vi "_HC_PM_and_temp.vi"(9 "PMavg":dbl=10.0, 10 "Bias_LO_equip":T1={"Node address"=19, "CAN Interface"="CAN1", "Cartridge band"=10, "Slave Node in"={"Address"=19, "Serial Number"=[16, 71, 55, 76, 1, 8, 0, -15]}, "ObjHandle out"=176554048, "POL"=1, "sb"=1, "GPIB_SM (SIS S,V)"="24", "GPIB_DMM (SIS I)"="22", "GPIB_SM (MAG I) "="25", "GPIB_SG(LO)"="19", "GPIB_PW (PAMP) "="6", "GPIB_TMP1(8ch)"="12", "GPIB_TMP2(2ch)  "="13", "WCA_avg"=10, "Rsen"=10.0, "BiasModule"=1, "LOModule "=5, "WCA_LO_FREQ_SET"={"YTO Low freq. [GHz]"=14.42, "YTO High freq. [GHz]"=17.7, "Kvco"=1, "Lock Pol."=0, "SET LO FREQ"=96.22222, "Multiplier"=6.0, "YTO (HEX)"=2014, "YTO ( FREQ)"=16.033167, "NULL PLL INTEGRATOR"=FALSE}, "Res for"=0} {"Res for" items=["none", "series res", "parallel res"]; "WCA_LO_FREQ_SET"."YTO ( FREQ)" min=25 max=150 step=0.0001 format="%.3f"; "WCA_LO_FREQ_SET"."Multiplier" min=3 max=6 step=3; "WCA_LO_FREQ_SET"."SET LO FREQ" min=25 max=150 step=0.0001 format="%.3f"; "WCA_LO_FREQ_SET"."Lock Pol." items=["Lower", "Upper"]; "WCA_LO_FREQ_SET"."Kvco" items=["7.5MHz/V", "15MHz/V"]; "WCA_LO_FREQ_SET"."YTO High freq. [GHz]" format="%.3f"; "WCA_LO_FREQ_SET"."YTO Low freq. [GHz]" format="%.3f"; "LOModule" items=["Manual Gunn+PAMP"=0, "PLL GUNN+PAMP"=5, "B10Lab LO"=1, "WCA LO"=2, ""=3, "YIG発信器"=4, "none"=99]; "BiasModule" items=["B10Lab Bias"=0, "WCA BiasModule"=1, "none"=99]; "Slave Node in"."Serial Number" format="%.0x"; "Slave Node in"."Address" format="%.0x"; "Cartridge band" max=10 step=1; "Node address" format="%.0x"}, 11 "Control":T2={"GPIB_ATT"="28", "6501Dev#"=1, "GPIB_SP"="18", "GPIB_PM"="13", "GPIB_DSA"="11", "GPIB_DMM (TPD)"="23", "GPIB_MPI"="2", "mortor設定"=[{"Axis"=0, "ID"=0, "HIspeed"=200.0, "LOspeed"=100.0, "ACCEL(ms)"=100.0, "Sratio"=50.0, "フリーラン\n"=FALSE, "文字列"="DSB HOT/COLD"}, {"Axis"=1, "ID"=0, "HIspeed"=4.0, "LOspeed"=4.0, "ACCEL(ms)"=100.0, "Sratio"=50.0, "フリーラン\n"=TRUE, "文字列"="SubMM Att"}, {"Axis"=0, "ID"=0, "HIspeed"=200.0, "LOspeed"=100.0, "ACCEL(ms)"=100.0, "Sratio"=50.0, "フリーラン\n"=TRUE, "文字列"="MPI Port1"}, {"Axis"=1, "ID"=0, "HIspeed"=200.0, "LOspeed"=100.0, "ACCEL(ms)"=100.0, "Sratio"=50.0, "フリーラン\n"=TRUE, "文字列"="MPI Port2"}], "DATAパス"=path "C:/Documents and Settings/?澤佳?/デスクトップ/data/プロトカ?トリッジ/100811_protC4-5/100904_P1_WCA_YIG", "DBパス "=path "Z:/band10/Labview_ALMA/MIX95/test", "comment"="100904_P1", "ColdCarts"="003601", "Th"=295.0, "Tc"=77.0, "Set_SIS_volt"=2.056451612903226, "Offset"=0.0, "control"=0, "FreqLO"=866.0, "Set_Mag_Cur"=800.0, "MPI offset(mm)"=22.986, "HOT/COLD"=0} {"HOT/COLD" items=["DSB", "SBR (Cart.)", "GainComp", "SBR (MIX)"]; "control" items=["CLOSE LOOP", "OPEN LOOP", "Not Control"]}) -> (3 "文字列":string="298.140000,297.760000,298.730000,304.990000,4.072000,4.151000,15.042000,80.446000,-19.064756,-17.597972,-30.625485,")   [LabVIEW 2017]
panel:
  # "LO freq. [GHz]"
  # "YTO LOW\n/High Freq."
  # "ZERO Intgrtr"
  # "Node Address"
  # "Serial Number"
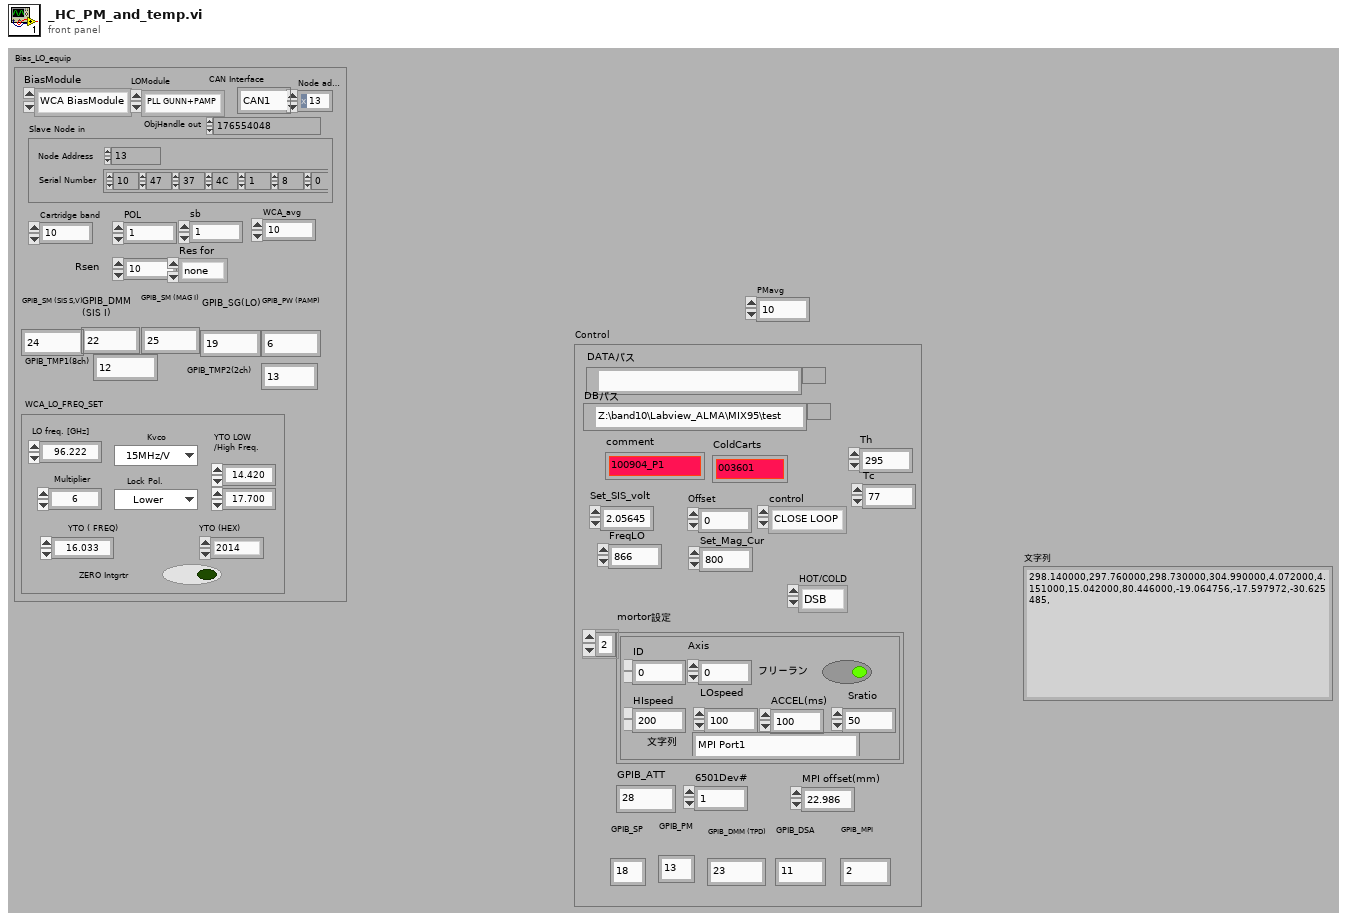
[diagram p1: front panel]
types:
  T1 = cluster{"Node address":u16, "CAN Interface":string, "Cartridge band":u32, "Slave Node in":cluster{"Address":i16, "Serial Number":i8[]}, "ObjHandle out":u32, "POL":u32, "sb":u32, "GPIB_SM (SIS S,V)":string, "GPIB_DMM (SIS I)":string, "GPIB_SM (MAG I) ":string, "GPIB_SG(LO)":string, "GPIB_PW (PAMP) ":string, "GPIB_TMP1(8ch)":string, "GPIB_TMP2(2ch)  ":string, "WCA_avg":i32, "Rsen":dbl, "BiasModule":u16, "LOModule ":u16, "WCA_LO_FREQ_SET":cluster{"YTO Low freq. [GHz]":sgl, "YTO High freq. [GHz]":sgl, "Kvco":u16, "Lock Pol.":u16, "SET LO FREQ":sgl, "Multiplier":sgl, "YTO (HEX)":u16, "YTO ( FREQ)":sgl, "NULL PLL INTEGRATOR":bool}, "Res for":u16}
  T2 = cluster{"GPIB_ATT":string, "6501Dev#":i16, "GPIB_SP":string, "GPIB_PM":string, "GPIB_DSA":string, "GPIB_DMM (TPD)":string, "GPIB_MPI":string, "mortor設定":cluster{"Axis":i16, "ID":i16, "HIspeed":dbl, "LOspeed":dbl, "ACCEL(ms)":dbl, "Sratio":dbl, "フリーラン\n":bool, "文字列":string}[], "DATAパス":path, "DBパス ":path, "comment":string, "ColdCarts":string, "Th":dbl, "Tc":dbl, "Set_SIS_volt":dbl, "Offset":dbl, "control":u16, "FreqLO":dbl, "Set_Mag_Cur":dbl, "MPI offset(mm)":dbl, "HOT/COLD":u16}
  T3 = cluster{"Axis":i16, "ID":i16, "HIspeed":dbl, "LOspeed":dbl, "ACCEL(ms)":dbl, "Sratio":dbl, "フリーラン\n":bool, "文字列":string}[]
  T4 = cluster{"Axis":i16, "ID":i16, "HIspeed":dbl, "LOspeed":dbl, "ACCEL(ms)":dbl, "Sratio":dbl, "フリーラン\n":bool, "文字列":string}
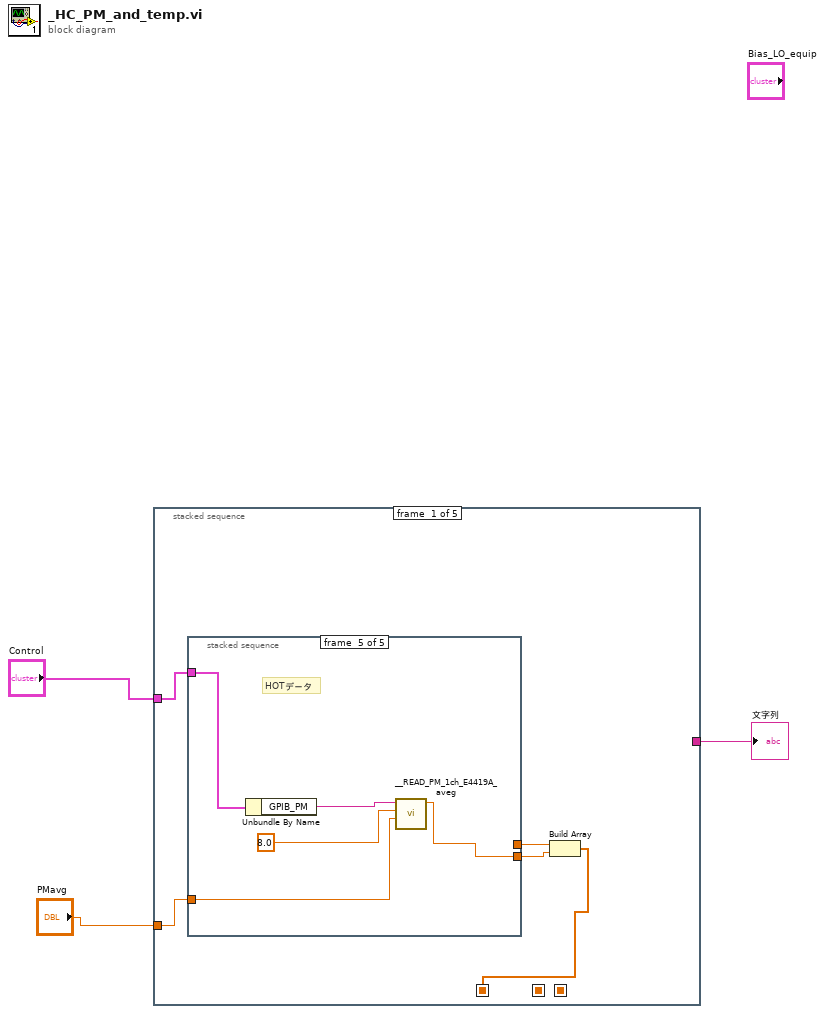
[diagram p0: block diagram]
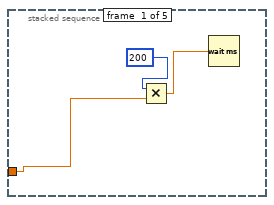
[diagram p2: hidden frame]
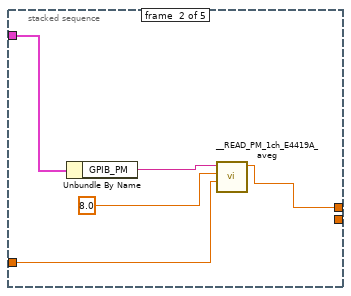
[diagram p3: hidden frame]
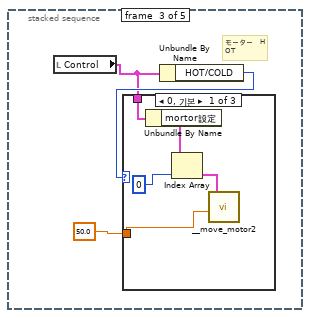
[diagram p4: hidden frame]
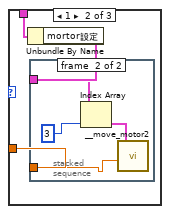
[diagram p5: hidden frame]
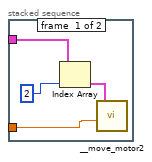
[diagram p6: hidden frame]
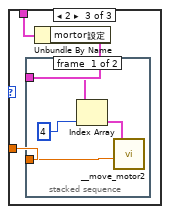
[diagram p7: hidden frame]
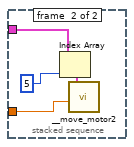
[diagram p8: hidden frame]
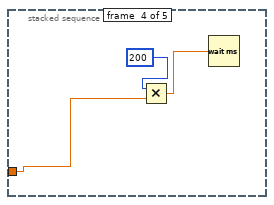
[diagram p9: hidden frame]
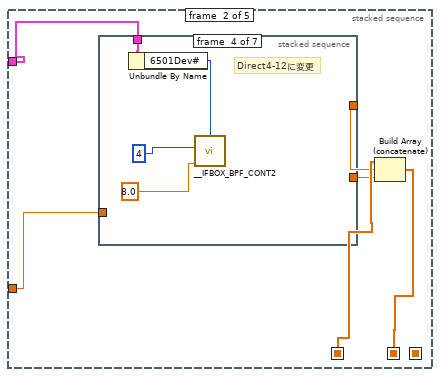
[diagram p10: hidden frame]
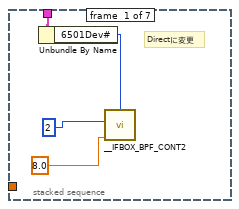
[diagram p11: hidden frame]
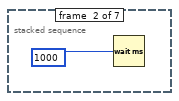
[diagram p12: hidden frame]
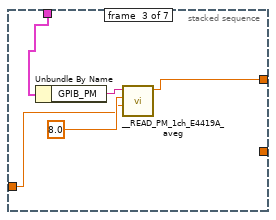
[diagram p13: hidden frame]
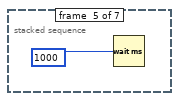
[diagram p14: hidden frame]
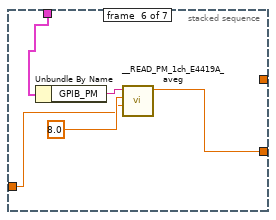
[diagram p15: hidden frame]
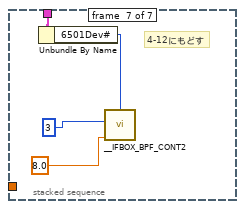
[diagram p16: hidden frame]
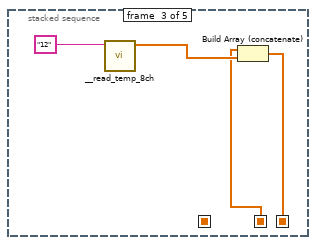
[diagram p17: hidden frame]
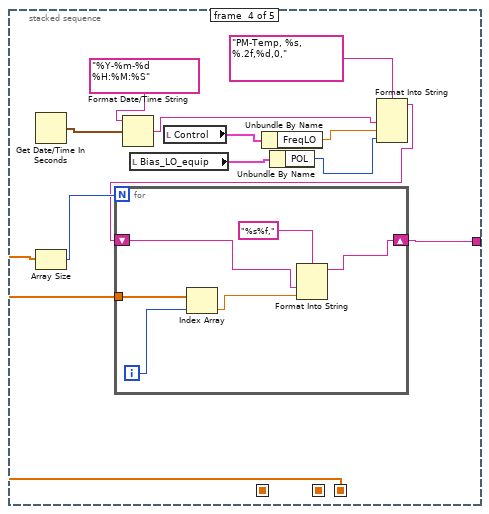
[diagram p18: hidden frame]
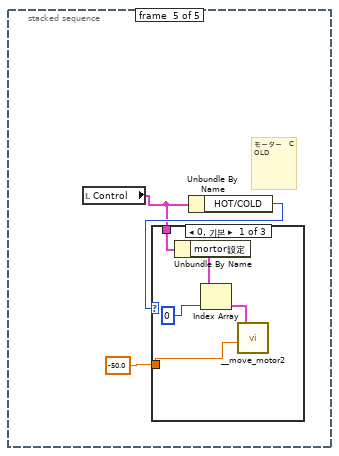
[diagram p19: hidden frame]
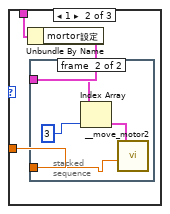
[diagram p20: hidden frame]
diagram:
  n1 = stacked-sequence {
    seq-local: [w4 _ _ _ _] -> [_ w57 _ _ _]
    seq-local: [_ w58 _ _ _] -> [_ _ w85 _ _]
    seq-local: [_ _ w86 _ _] -> [_ _ _ w89 _]
    tunnel: "Control" -> [w8 w60 _ _ _]
    tunnel: "PMavg" -> [w7 w59 _ _ _]
    tunnel: [_ _ _ w99 _] -> w1
    frame #0 {
      n2 = stacked-sequence {
        tunnel: w8 -> [_ w15 _ _ w53]
        tunnel: w7 -> [w9 w13 _ w47 w51]
        tunnel: [_ w12 _ _ _] -> w6
        tunnel: [_ _ _ _ w50] -> w5
        frame #0 {
          n3 = Multiply(x=200, y=w9) -> (x*y=w11:dbl)
          n4 = Wait (ms)(milliseconds to wait=w11) -> ()  [unwired: 1 out]
        }
        frame #1 {
          n5 = Unbundle By Name(w15) -> ("GPIB_PM"=w16:string)
          n6 = call "__READ_PM_1ch_E4419A_aveg.VI"("aveg"=w13, "frq(GHz)"=8.0, "GPIB"=w16) -> ("chA"=w12:dbl)  [unwired: 4 in]
        }
        frame #2 {
          # "モーター　HOT"
          n7 = local read "Control"() -> (w17:T2)
          n8 = Unbundle By Name(w17) -> ("HOT/COLD"=w18:u16)
          n9 = case shown="0, 기본" w18 {
            tunnel: w17 -> [w23 w27 w38]
            tunnel: 50.0 -> [w20 w25 w36]
            frame 0, Default {
              n10 = Unbundle By Name(w23) -> ("mortor設定"=w22:T3)
              n11 = Index Array(array=w22, index=0) -> (element=w21:T4)
              n12 = call "__move_motor2.vi"("Moving distance"=w20, "motor setup"=w21) -> ()  [unwired: 2 in, 2 out]
            }
            frame 1 {
              n13 = Unbundle By Name(w27) -> ("mortor設定"=w26:T3)
              n14 = stacked-sequence {
                tunnel: w26 -> [w30 w34]
                tunnel: w25 -> [w28 w32]
                frame #0 {
                  n15 = Index Array(array=w30, index=2) -> (element=w29:T4)
                  n16 = call "__move_motor2.vi"("Moving distance"=w28, "motor setup"=w29) -> ()  [unwired: 2 in, 2 out]
                }
                frame #1 {
                  n17 = Index Array(array=w34, index=3) -> (element=w33:T4)
                  n18 = call "__move_motor2.vi"("Moving distance"=w32, "motor setup"=w33) -> ()  [unwired: 2 in, 2 out]
                }
              }
            }
            frame 2 {
              n19 = Unbundle By Name(w38) -> ("mortor設定"=w37:T3)
              n20 = stacked-sequence {
                tunnel: w37 -> [w41 w45]
                tunnel: w36 -> [w39 w43]
                frame #0 {
                  n21 = Index Array(array=w41, index=4) -> (element=w40:T4)
                  n22 = call "__move_motor2.vi"("Moving distance"=w39, "motor setup"=w40) -> ()  [unwired: 2 in, 2 out]
                }
                frame #1 {
                  n23 = Index Array(array=w45, index=5) -> (element=w44:T4)
                  n24 = call "__move_motor2.vi"("Moving distance"=w43, "motor setup"=w44) -> ()  [unwired: 2 in, 2 out]
                }
              }
            }
          }
        }
        frame #3 {
          n25 = Multiply(x=200, y=w47) -> (x*y=w49:dbl)
          n26 = Wait (ms)(milliseconds to wait=w49) -> ()  [unwired: 1 out]
        }
        frame #4 {
          # "HOTデータ"
          n27 = Unbundle By Name(w53) -> ("GPIB_PM"=w54:string)
          n28 = call "__READ_PM_1ch_E4419A_aveg.VI"("aveg"=w51, "frq(GHz)"=8.0, "GPIB"=w54) -> ("chA"=w50:dbl)  [unwired: 4 in]
        }
      }
      n29 = Build Array(w6, w5) -> (w4:dbl[])
    }
    frame #1 {
      n30 = stacked-sequence {
        tunnel: w60 -> [w64 _ w66 w74 _ w77 w84]
        tunnel: w59 -> [_ _ w68 _ _ w78 _]
        tunnel: [_ _ w67 _ _ _ _] -> w56
        tunnel: [_ _ _ _ _ w76 _] -> w55
        frame #0 {
          # "Directに変更"
          n31 = Unbundle By Name(w64) -> ("6501Dev#"=w63:i16)
          n32 = call "__IFBOX_BPF_CONT2.vi"("YIG frq(GHz) 2"=8.0, "フィルター（1:YIG,2:direct,3:4-12BPF,4:direct4-12BPF）"=2, "Dev#"=w63) -> ()  [unwired: 1 in]
        }
        frame #1 {
          n33 = Wait (ms)(milliseconds to wait=1000) -> ()  [unwired: 1 out]
        }
        frame #2 {
          n34 = Unbundle By Name(w66) -> ("GPIB_PM"=w70:string)
          n35 = call "__READ_PM_1ch_E4419A_aveg.VI"("aveg"=w68, "frq(GHz)"=8.0, "GPIB"=w70) -> ("chA"=w67:dbl)  [unwired: 4 in]
        }
        frame #3 {
          # "Direct4-12に変更"
          n36 = Unbundle By Name(w74) -> ("6501Dev#"=w73:i16)
          n37 = call "__IFBOX_BPF_CONT2.vi"("YIG frq(GHz) 2"=8.0, "フィルター（1:YIG,2:direct,3:4-12BPF,4:direct4-12BPF）"=4, "Dev#"=w73) -> ()  [unwired: 1 in]
        }
        frame #4 {
          n38 = Wait (ms)(milliseconds to wait=1000) -> ()  [unwired: 1 out]
        }
        frame #5 {
          n39 = Unbundle By Name(w77) -> ("GPIB_PM"=w80:string)
          n40 = call "__READ_PM_1ch_E4419A_aveg.VI"("aveg"=w78, "frq(GHz)"=8.0, "GPIB"=w80) -> ("chA"=w76:dbl)  [unwired: 4 in]
        }
        frame #6 {
          # "4-12にもどす"
          n41 = Unbundle By Name(w84) -> ("6501Dev#"=w83:i16)
          n42 = call "__IFBOX_BPF_CONT2.vi"("YIG frq(GHz) 2"=8.0, "フィルター（1:YIG,2:direct,3:4-12BPF,4:direct4-12BPF）"=3, "Dev#"=w83) -> ()  [unwired: 1 in]
        }
      }
      n43 = Build Array (concatenate)(w57, w56, w55) -> (w58:dbl[])
    }
    frame #2 {
      n44 = call "__read_temp_8ch.vi"("GIPB番号"="12") -> ("配列"=w87:dbl[])  [unwired: 10 in]
      n45 = Build Array (concatenate)(w85, w87) -> (w86:dbl[])
    }
    frame #3 {
      n46 = Get Date/Time In Seconds() -> (seconds since 1Jan1904=w95:timestamp)
      n47 = Array Size(array=w89) -> (size(s)=w100:i32)
      n48 = Format Date/Time String(time format string (%c)="%Y-%m-%d  %H:%M:%S", seconds (now)=w95) -> (date/time string=w93:string)  [unwired: 1 in]
      n49 = local read "Bias_LO_equip"() -> (w98:T1)
      n50 = local read "Control"() -> (w97:T2)
      n51 = Unbundle By Name(w97) -> ("FreqLO"=w92:dbl)
      n52 = Unbundle By Name(w98) -> ("POL"=w91:u32)
      n53 = Format Into String(format string="PM-Temp, %s, %.2f,%d,0,", w93, w92, w91) -> (resulting string=w90:string)  [unwired: 2 in, 1 out]
      n54 = for {
        N: w100 -> [_]
        shift-right: [w103] -> w99
        shift-left: w90 -> [w104]
        tunnel: w89 -> [w102]
        i -> [w106]
        n55 = Index Array(array=w102, index=w106) -> (element=w101:dbl)
        n56 = Format Into String(format string="%s%f,", w104, w101) -> (resulting string=w103:string)  [unwired: 2 in, 1 out]
      }
    }
    frame #4 {
      # "モーター　COLD"
      n57 = local read "Control"() -> (w107:T2)
      n58 = Unbundle By Name(w107) -> ("HOT/COLD"=w108:u16)
      n59 = case shown="0, 기본" w108 {
        tunnel: w107 -> [w113 w117 w128]
        tunnel: -50.0 -> [w110 w115 w126]
        frame 0, Default {
          n60 = Unbundle By Name(w113) -> ("mortor設定"=w112:T3)
          n61 = Index Array(array=w112, index=0) -> (element=w111:T4)
          n62 = call "__move_motor2.vi"("Moving distance"=w110, "motor setup"=w111) -> ()  [unwired: 2 in, 2 out]
        }
        frame 1 {
          n63 = Unbundle By Name(w117) -> ("mortor設定"=w116:T3)
          n64 = stacked-sequence {
            tunnel: w116 -> [w120 w124]
            tunnel: w115 -> [w118 w122]
            frame #0 {
              n65 = Index Array(array=w120, index=2) -> (element=w119:T4)
              n66 = call "__move_motor2.vi"("Moving distance"=w118, "motor setup"=w119) -> ()  [unwired: 2 in, 2 out]
            }
            frame #1 {
              n67 = Index Array(array=w124, index=3) -> (element=w123:T4)
              n68 = call "__move_motor2.vi"("Moving distance"=w122, "motor setup"=w123) -> ()  [unwired: 2 in, 2 out]
            }
          }
        }
        frame 2 {
          n69 = Unbundle By Name(w128) -> ("mortor設定"=w127:T3)
          n70 = stacked-sequence {
            tunnel: w127 -> [w131 w135]
            tunnel: w126 -> [w129 w133]
            frame #0 {
              n71 = Index Array(array=w131, index=4) -> (element=w130:T4)
              n72 = call "__move_motor2.vi"("Moving distance"=w129, "motor setup"=w130) -> ()  [unwired: 2 in, 2 out]
            }
            frame #1 {
              n73 = Index Array(array=w135, index=5) -> (element=w134:T4)
              n74 = call "__move_motor2.vi"("Moving distance"=w133, "motor setup"=w134) -> ()  [unwired: 2 in, 2 out]
            }
          }
        }
      }
    }
  }
  "文字列" <- w1
